vi "interpret_36bytes (SubVI).vi"(11 "data in":string) -> (0 "low cell, V":sgl, 1 "high cell, V":sgl, 2 "Amps":sgl, 3 "Volts":sgl, 4 "difference, V":sgl format="%_3g")   [LabVIEW 2018]
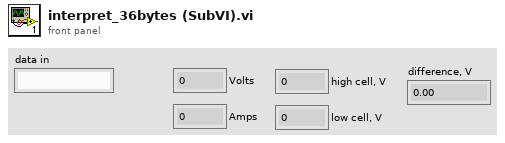
[diagram p1: front panel]
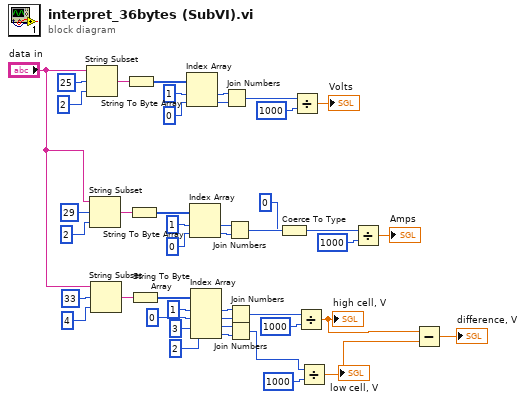
[diagram p0: block diagram]
diagram:
  n1 = String Subset(string="data in", offset (0)=25, length (rest)=2 ("length (rest)")) -> (substring=w32:string)
  n2 = String Subset(string="data in", offset (0)=29, length (rest)=2 ("length (rest)")) -> (substring=w31:string)
  n3 = String Subset(string="data in", offset (0)=33, length (rest)=4 ("length (rest)")) -> (substring=w20:string)
  n4 = String To Byte Array(string=w32) -> (unsigned byte array=w38:u8[])
  n5 = String To Byte Array(string=w31) -> (unsigned byte array=w30:u8[])
  n6 = String To Byte Array(string=w20) -> (unsigned byte array=w17:u8[])
  n7 = Index Array(array=w38, index #1=1 ("index"), index #2=0 ("index")) -> (element #1=w42:u8, element #2=w41:u8)
  n8 = Index Array(array=w30, index #1=1 ("index"), index #2=0 ("index")) -> (element #1=w27:u8, element #2=w26:u8)
  n9 = Index Array(array=w17, index #1=1 ("index"), index #2=0 ("index"), index #3=3 ("index"), index #4=2 ("index")) -> (element #1=w13:u8, element #2=w14:u8, element #3=w7:u8, element #4=w6:u8)
  n10 = Join Numbers(hi=w42, lo=w41) -> ((hi.lo)=w37:u16)
  n11 = Join Numbers(hi=w27, lo=w26) -> ((hi.lo)=w23:u16)
  n12 = Join Numbers(hi=w13, lo=w14) -> ((hi.lo)=w18:u16)
  n13 = Join Numbers(hi=w7, lo=w6) -> ((hi.lo)=w4:u16)
  n14 = Coerce To Type(0:w23, 1:i16 0 ("y")) -> (2:w21:i16)
  n15 = Divide(x=w37, y=u16 1000) -> (x/y=→"Volts":dbl)
  n16 = Divide(x=w18, y=u16 1000) -> (x/y=w3:sgl)
  "high cell, V" <- w3
  n17 = Divide(x=w4, y=u16 1000) -> (x/y=w2:sgl)
  "low cell, V" <- w2
  n18 = Divide(x=w21, y=u16 1000) -> (x/y=→"Amps":dbl)
  n19 = Subtract(x=w3, y=w2) -> (x-y=→"difference, V":sgl)
